vi "Flussdichte Anpassen.vi"(0 "VISA Name FG in(FG)":refnum<visa-resource-name>="USB0::0x0957::0x0407::MY44043889::INSTR", 5 "VISA Name OZ In (OZ)":refnum<visa-resource-name>="USB0::0x0957::0x179B::MY54313507::INSTR", 7 "max_spg_fg":dbl format="%#_13g", 9 "min_spg_fg":dbl format="%#_13g", 11 "Error_in":errorcluster) -> (2 "spg_abw":dbl format="%#_13g", 4 "VISA Name FG out":refnum<visa-resource-name>="USB0::0x0957::0x0407::MY44043889::INSTR", 6 "VISA Name OZ Out":refnum<visa-resource-name>="USB0::0x0957::0x179B::MY54313507::INSTR", 8 "Output H-Array":dbl[](array[numeric]), 10 "Output B-Array":dbl[](array[numeric]), 13 "b_gew":dbl format="%#_13g", 15 "Error_out":errorcluster)   [LabVIEW 2016]
panel:
  out "i":i32
  out "spg":dbl format="%#_13g"
  out "add":dbl format="%#_13g"
  in  "Abbrechen":bool
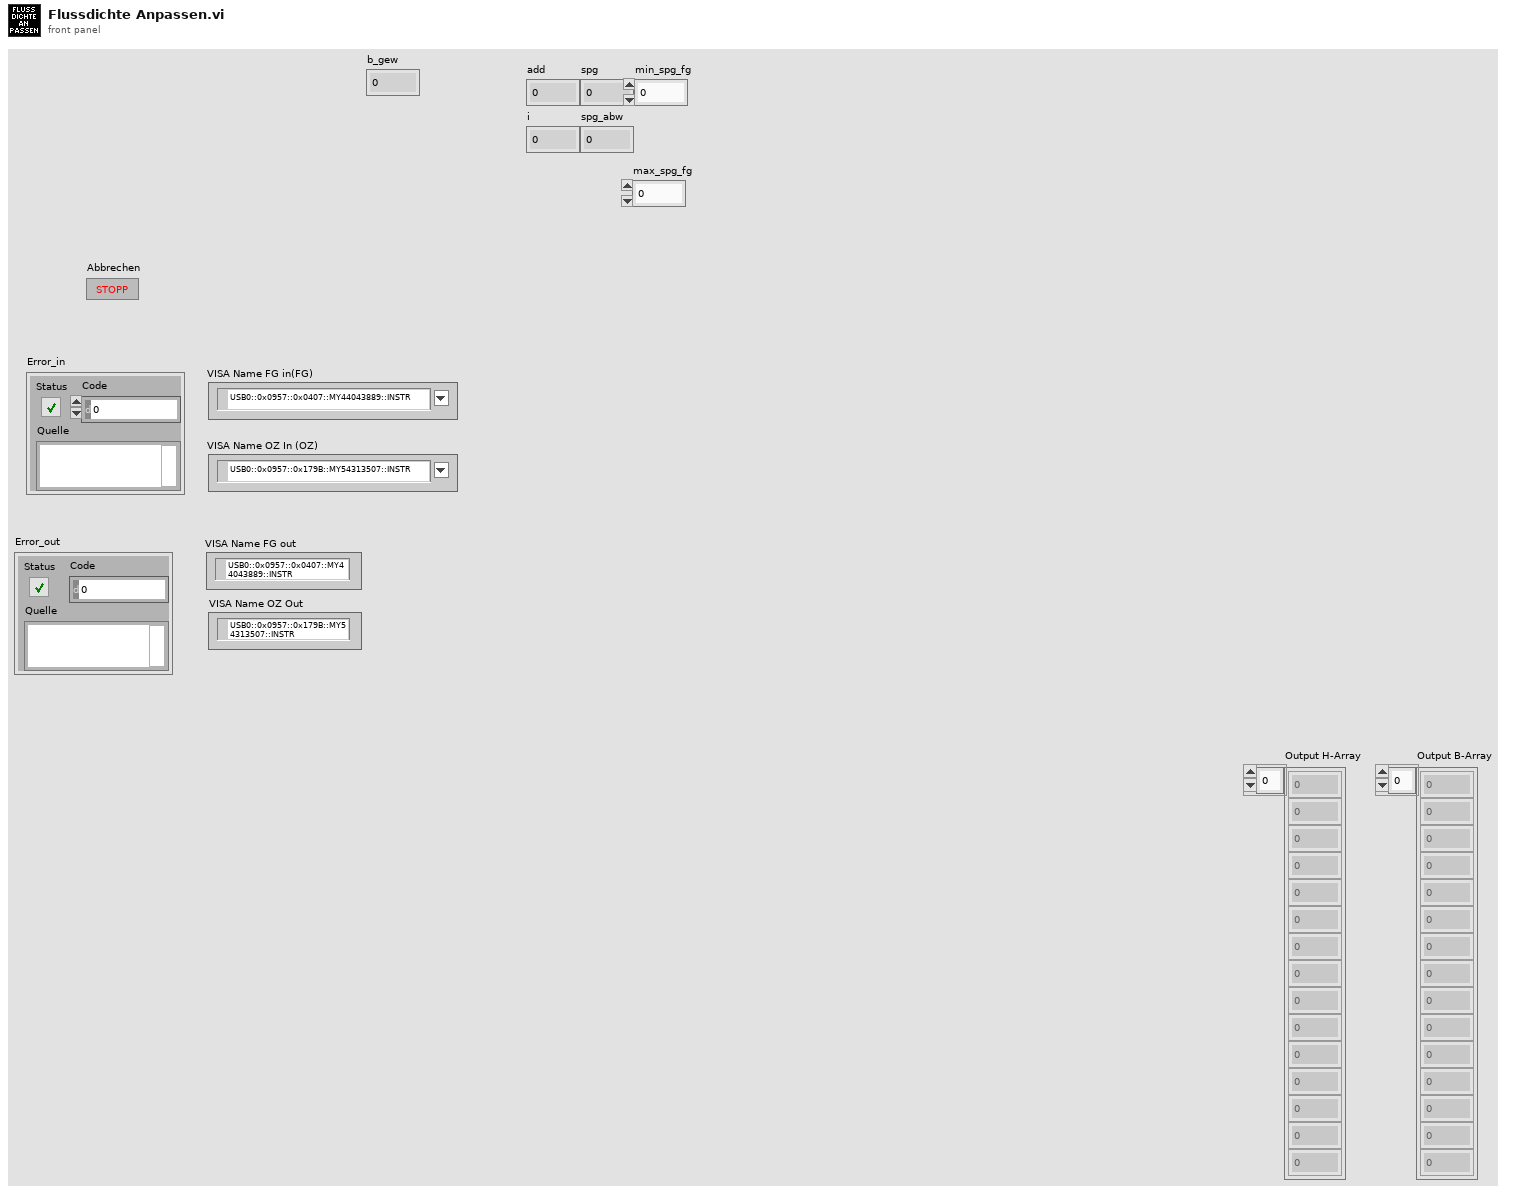
[diagram p1: front panel]
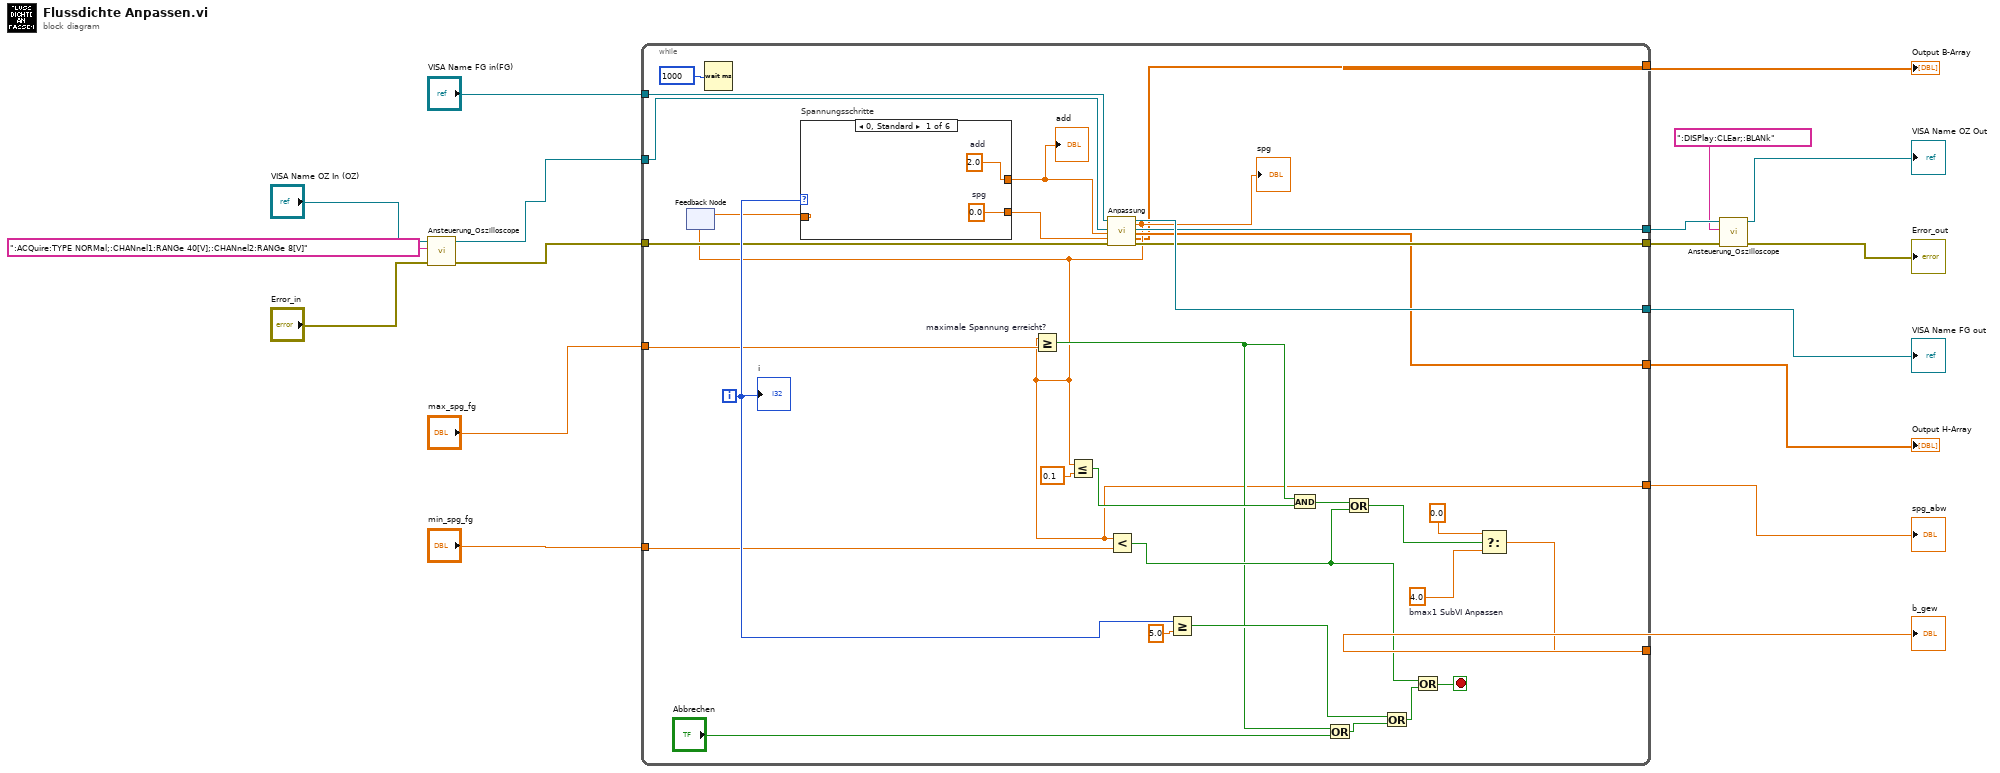
[diagram p0: block diagram]
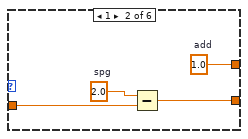
[diagram p2: hidden frame]
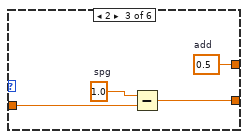
[diagram p3: hidden frame]
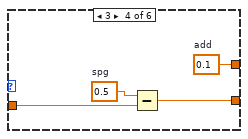
[diagram p4: hidden frame]
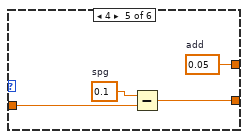
[diagram p5: hidden frame]
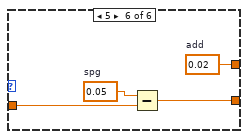
[diagram p6: hidden frame]
diagram:
  n1 = call "Ansteuerung_Oszilloscope.vi"("Error_in"="Error_in", "Eingangs-String"=":ACQuire:TYPE NORMal;:CHANnel1:RANGe 40[V];:CHANnel2:RANGe 8[V]", "VISA Name OZ in(OZ)"="VISA Name OZ In (OZ)") -> ("Error_out"=w3:errorcluster, "VISA Name OZ out"=w5:refnum<visa-resource-name>)  [unwired: 6 in, 1 out]
  n2 = while {
    tunnel: "min_spg_fg" -> [w45]
    tunnel: [w20] -> w17
    tunnel: [w35] -> w9
    tunnel: w3 -> [w41]
    tunnel: [w37] -> w16
    tunnel: "VISA Name FG in(FG)" -> [w40]
    tunnel: [w36] -> w11
    tunnel: w5 -> [w39]
    tunnel: "max_spg_fg" -> [w33]
    tunnel: [w19] -> w13
    tunnel: [w34] -> w12
    tunnel: [w22] -> w6
    i -> [w47]
    stop <- w43 stop-if-true
    w26 = 4.0  # bmax1 SubVI Anpassen
    n3 = feedback #1() -> (w21:dbl)  [unwired: 1 in]
    n4 = Wait (ms)(milliseconds to wait=1000) -> ()  [unwired: 1 out]
    n5 = case "Spannungsschritte" shown="0, Standard" w47 {
      tunnel: [w50 w52 w57 w61 w65 w69] -> w38
      tunnel: [w51 w53 w56 w60 w64 w68] -> w31
      tunnel: w21 -> [_ w54 w58 w62 w66 w70]
      frame 0, Default {
        w50 = 0.0  # spg
        w51 = 2.0  # add
      }
      frame 1 {
        w55 = 2.0  # spg
        w53 = 1.0  # add
        n6 = Subtract(x=w55, y=w54) -> (x-y=w52:dbl)
      }
      frame 2 {
        w59 = 1.0  # spg
        w56 = 0.5  # add
        n7 = Subtract(x=w59, y=w58) -> (x-y=w57:dbl)
      }
      frame 3 {
        w63 = 0.5  # spg
        w60 = 0.1  # add
        n8 = Subtract(x=w63, y=w62) -> (x-y=w61:dbl)
      }
      frame 4 {
        w67 = 0.1  # spg
        w64 = 0.05  # add
        n9 = Subtract(x=w67, y=w66) -> (x-y=w65:dbl)
      }
      frame 5 {
        w71 = 0.05  # spg
        w68 = 0.02  # add
        n10 = Subtract(x=w71, y=w70) -> (x-y=w69:dbl)
      }
    }
    "add" <- w31
    n11 = call "Anpassung.vi"("VISA Name FG in(FG)"=w40, "VISA Name OZ In (OZ)"=w39, "Add (0)"=w31, "Spg (0)"=w38, "Error_in"=w41) -> ("VISA Name FG out"=w37:refnum<visa-resource-name>, "Spg_new_out"=w20:dbl, "VISA Name OZ Out"=w36:refnum<visa-resource-name>, "Output H-Array"=w34:dbl[], "Output B-Array"=w19:dbl[], "Error_out"=w35:errorcluster)  [unwired: 8 in, 1 out]
    "spg" <- w20
    n12 = feedback-in #1(w20) -> ()
    n13 = Greater Or Equal? "maximale Spannung erreicht?"(x=w20, y=w33) -> (x >= y?=w23:bool)
    n14 = Less Or Equal?(x=w20, y=0.1) -> (x <= y?=w24:bool)
    n15 = Less?(x=w20, y=w45) -> (x < y?=w25:bool)
    n16 = Greater Or Equal?(x=w47, y=5.0) -> (x >= y?=w48:bool)
    n17 = And(x=w23, y=w24) -> (x .and. y?=w27:bool)
    n18 = Or(x=w23, y="Abbrechen") -> (x .or. y?=w49:bool)
    n19 = Or(x=w27, y=w25) -> (x .or. y?=w28:bool)
    n20 = Or(x=w48, y=w49) -> (x .or. y?=w44:bool)
    n21 = Or(x=w25, y=w44) -> (x .or. y?=w43:bool)
    n22 = Select(t=0.0 ("bmax1"), s=w28, f=w26) -> (s? t:f=w22:dbl)
    "i" <- w47
  }
  "spg_abw" <- w17
  "VISA Name FG out" <- w16
  "Output B-Array" <- w13
  "Output H-Array" <- w12
  "b_gew" <- w6
  n23 = call "Ansteuerung_Oszilloscope.vi"("Error_in"=w9, "Eingangs-String"=":DISPlay:CLEar;:BLANk", "VISA Name OZ in(OZ)"=w11) -> ("Error_out"=→"Error_out":errorcluster, "VISA Name OZ out"=→"VISA Name OZ Out":refnum<visa-resource-name>)  [unwired: 6 in, 1 out]
